vi "calibration.vi"(8 "error in (no error)":errorcluster, 10 "Pram_calib In":T1, 11 "Spectrum In":i64[](array[numeric])) -> (0 "Error Out":errorcluster, 1 "set max":cluster{"Channels":dbl[], "Intensity":dbl[]}, 2 "Param Calibrazione":T1, 3 "Spectrum Out":T3)   [LabVIEW 2023]
uses:
  control/calib.ctl
  control/param_calibrazione.ctl
  <vilib>/Analysis/1siggen.llb/Ramp Pattern by Samples.vi
  <vilib>/Utility/file.llb/Read Delimited Spreadsheet (string).vi
  control/global name path.vi
  <vilib>/Utility/file.llb/Write Delimited Spreadsheet (DBL).vi
  <vilib>/Utility/file.llb/Read Delimited Spreadsheet (DBL).vi
  queue/Front Panel Message Queue.lvlib
  <vilib>/Analysis/NI_AALBase.lvlib
panel:
  in  "load_spct":bool
  in  "save_spct":bool
  out "Load Param Calib":T1
  in  "load_param":bool
  in  "save_param":bool
  out "peaks found":i32
  out "Spectrum Init":T2(graph)
  in  "side points":i32=19
  in  "polynomial order":i32=9
  in  "Max Channel":i32=5800
  in  "Min Channel":i32=500
  in  "width":i32=60 min=3
  in  "threshold":dbl=50.0 format="%0.2f"
  out "Spectrum Calibrated":cluster{dbl[], dbl[]}(graph)
  in  "list_peak_energies":string[][](array[string])
  out "Calibration":cluster{dbl[], dbl[]}[](graph)
  in  "List Calibration":T4[](array[typedef]) {"Select Line" items=["Ka1", "Ka2", "Kb1", "La1", "La2", "Lb1", "Lb2", "Lg1"]; "Select Element" items=["Li", "Be", "B", "C", "N", "O", "F", "Ne", "Na", "Mg", "Al", "Si", "P", "S", "Cl", "Ar", "K", "Ca", "Sc", "Ti", "V", "Cr", "Mn", "Fe", "Co", "Ni", "Cu", "Zn", "Ga", "Ge", "As", "Se", "Br", "Kr", "Rb", "Sr", "Y", "Zr", "Nb", "Mo", "Tc", "Ru", "Rh", "Pd", "Ag", "Cd", "In", "Sn", "Sb", "Te", "I", "Xe", "Cs", "Ba", "La", "Ce", "Pr", "Nd", "Pm", "Sm", "Eu", "Gd", "Tb", "Dy", "Ho", "Er", "Tm", "Yb", "Lu", "Hf", "Ta", "W", "Re", "Os", "Ir", "Pt", "Au", "Hg", "Tl", "Pb", "Bi", "Po", "At", "Rn", "Fr", "Ra", "Ac", "Th", "Pa", "U", "Np", "Pu", "Am"]}
  in  "back":bool
  out "Spectrum Analyzed":cluster{"Channels":dbl[], "Intensity":dbl[]}[](graph)
  in  "smooth":bool
  in  "peak":bool
  in  "Stop Button":bool
  in  "Select Line":u16(ring) items=["Ka1", "Ka2", "Kb1", "La1", "La2", "Lb1", "Lb2", "Lg1"]
  in  "Select Element":u16(ring) items=["Li", "Be", "B", "C", "N", "O", "F", "Ne", "Na", "Mg", "Al", "Si", "P", "S", "Cl", "Ar", "K", "Ca", "Sc", "Ti", "V", "Cr", "Mn", "Fe", "Co", "Ni", "Cu", "Zn", "Ga", "Ge", "As", "Se", "Br", "Kr", "Rb", "Sr", "Y", "Zr", "Nb", "Mo", "Tc", "Ru", "Rh", "Pd", "Ag", "Cd", "In", "Sn", "Sb", "Te", "I", "Xe", "Cs", "Ba", "La", "Ce", "Pr", "Nd", "Pm", "Sm", "Eu", "Gd", "Tb", "Dy", "Ho", "Er", "Tm", "Yb", "Lu", "Hf", "Ta", "W", "Re", "Os", "Ir", "Pt", "Au", "Hg", "Tl", "Pb", "Bi", "Po", "At", "Rn", "Fr", "Ra", "Ac", "Th", "Pa", "U", "Np", "Pu", "Am"]
  # "Smooth Parameters"
  # "Search Peak Parameter"
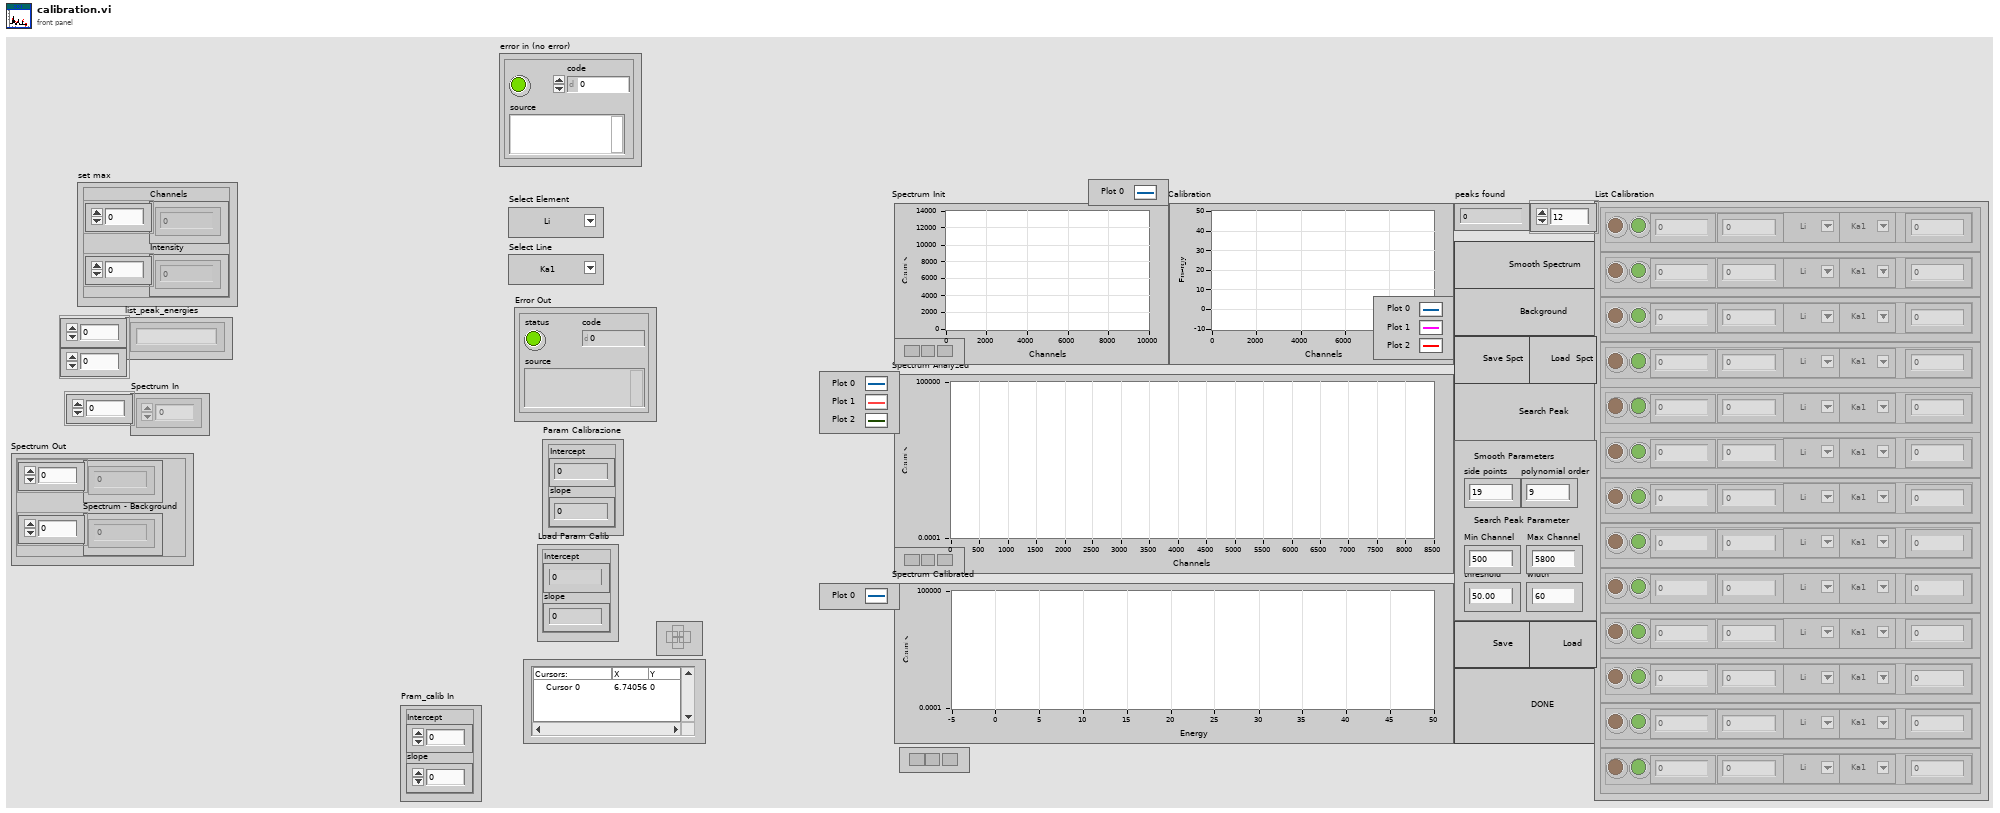
[diagram p1: front panel]
types:
  T1 = typedef "param_calibrazione.ctl" = cluster{"Intercept":dbl, "slope":dbl}
  T2 = cluster{"Ramp Pattern":dbl[], "Spectrum In":i64[]}
  T3 = cluster{"Array":dbl[], "Spectrum - Background":dbl[]}
  T4 = typedef "calib.ctl" = cluster{"select":bool, "Position":dbl, "Select Element":u16, "Select Line":u16, "Intensity":dbl, "Energy":dbl, "best":bool}
  T5 = typedef "Front Panel Message Queue.lvlib/Calibrazione Message Queues.ctl" = cluster{"Main":refnum<queue>, "Data":refnum<queue>}
  T6 = cluster{"Position":dbl[], "Intensity":dbl[], "Energy":dbl[]}
  T7 = cluster{"Ramp Pattern":dbl[], "Smoothed Spectrum":dbl[]}
  T8 = cluster{"Ramp Pattern":dbl[], "Spectrum - Background":dbl[]}
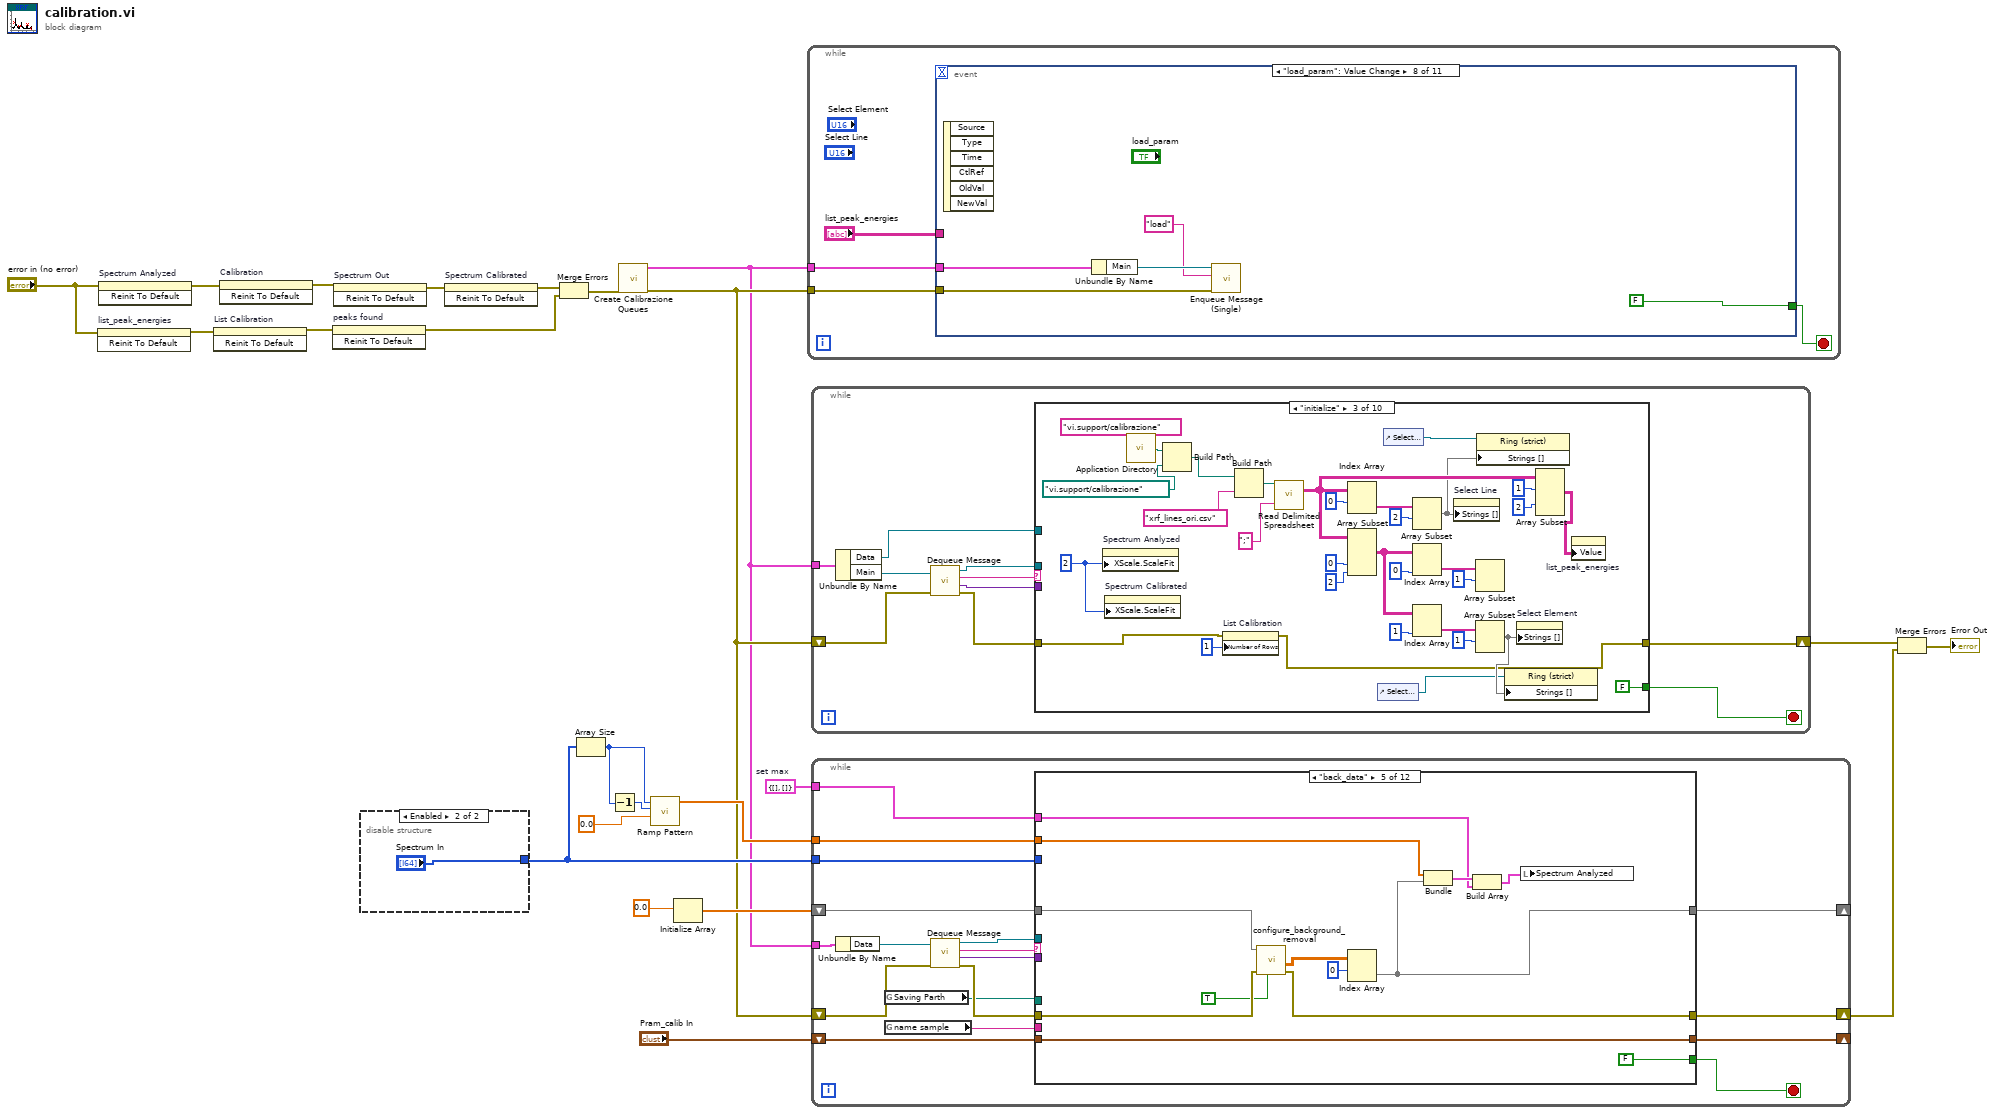
[diagram p0: block diagram]
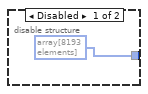
[diagram p2: hidden frame]
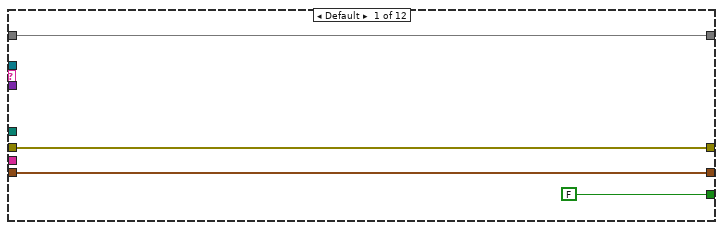
[diagram p3: hidden frame]
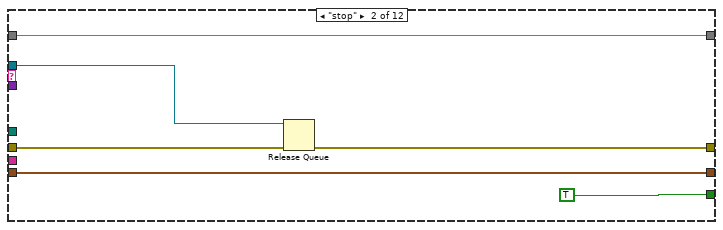
[diagram p4: hidden frame]
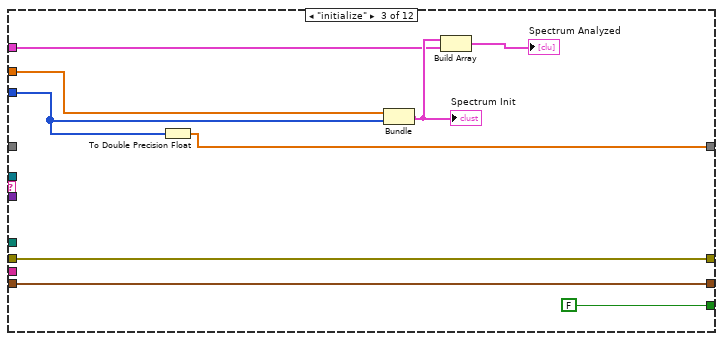
[diagram p5: hidden frame]
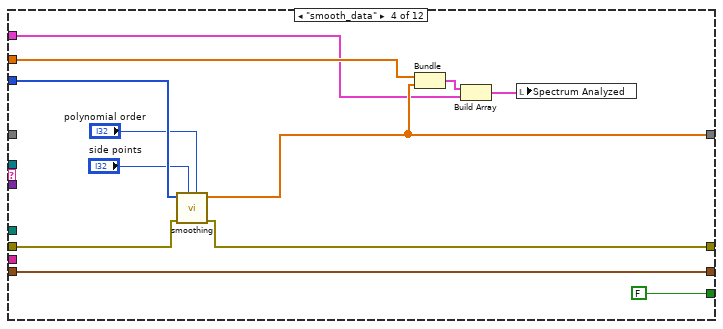
[diagram p6: hidden frame]
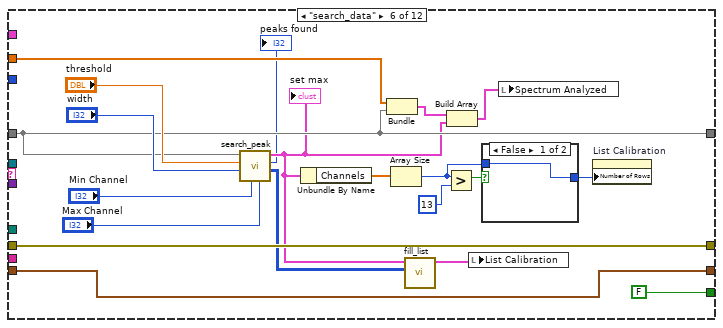
[diagram p7: hidden frame]
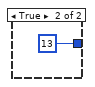
[diagram p8: hidden frame]
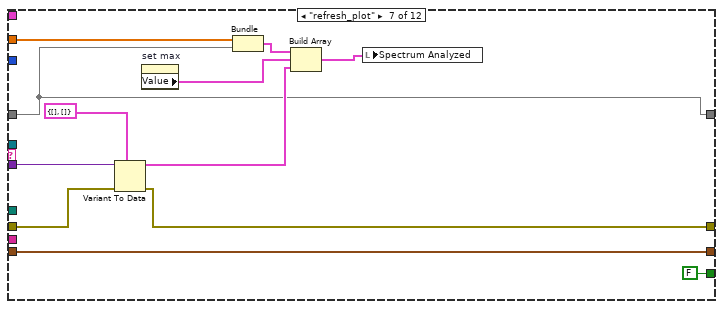
[diagram p9: hidden frame]
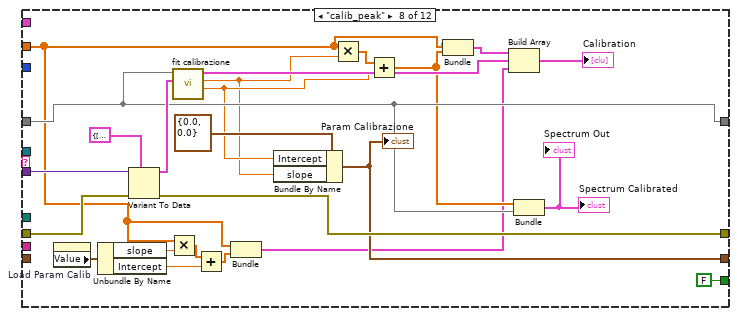
[diagram p10: hidden frame]
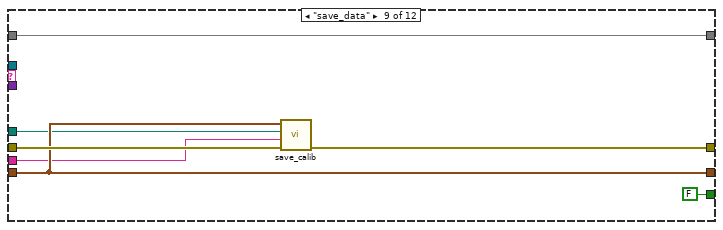
[diagram p11: hidden frame]
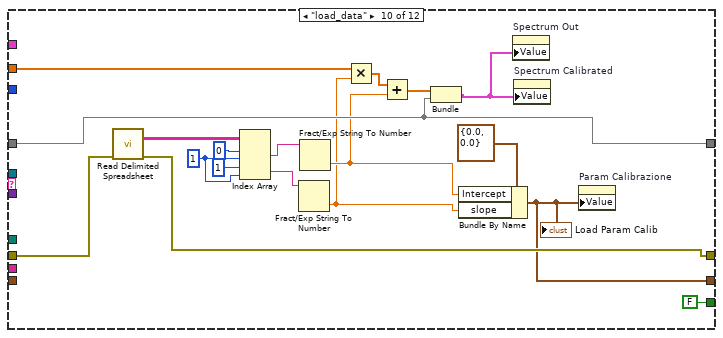
[diagram p12: hidden frame]
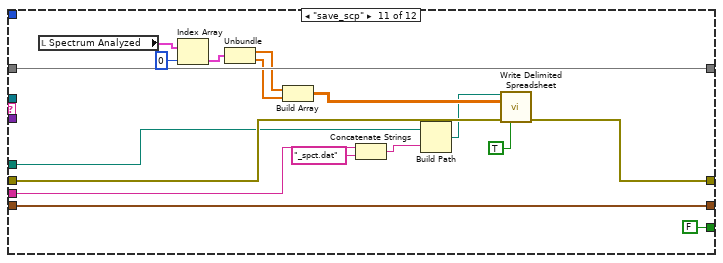
[diagram p13: hidden frame]
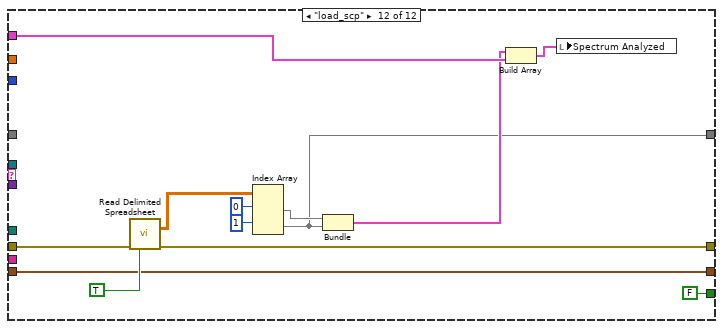
[diagram p14: hidden frame]
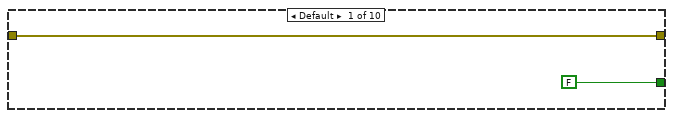
[diagram p15: hidden frame]
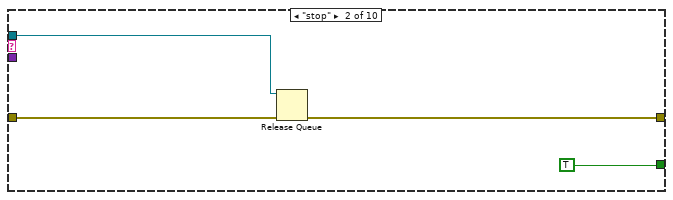
[diagram p16: hidden frame]
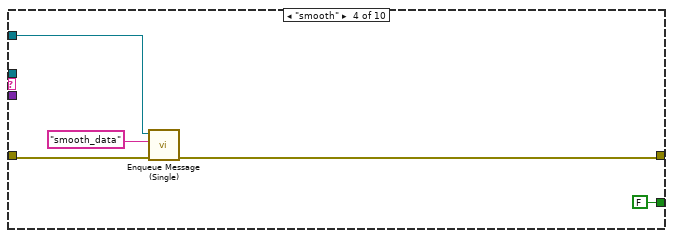
[diagram p17: hidden frame]
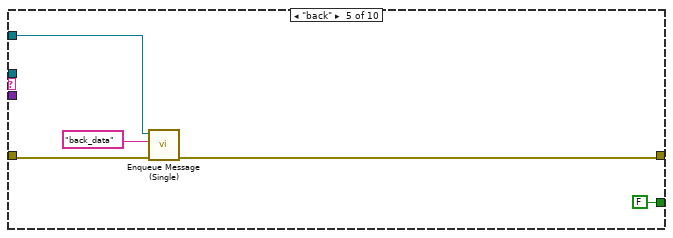
[diagram p18: hidden frame]
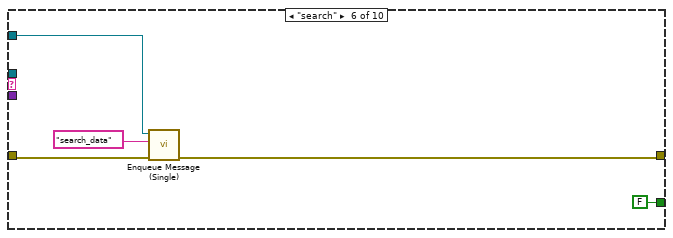
[diagram p19: hidden frame]
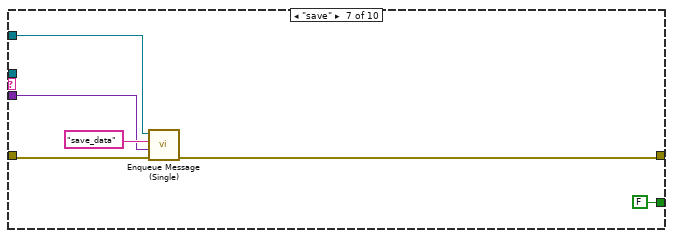
[diagram p20: hidden frame]
diagram:
  w16 = cluster{"Channels":dbl[], "Intensity":dbl[]} {"Channels"=[], "Intensity"=[]}  # set max
  n1 = invoke on="list_peak_energies" class="Arr (strict)" method="Reinit To Default"(error in="error in (no error)") -> (error out=w11:errorcluster)  [unwired: 2 in, 2 out]
  n2 = invoke on="Spectrum Analyzed" class="XYGraph (strict)" method="Reinit To Default"(error in="error in (no error)") -> (error out=w13:errorcluster)  [unwired: 2 in, 2 out]
  n3 = invoke on="List Calibration" class="Arr (strict)" method="Reinit To Default"(error in=w11) -> (error out=w9:errorcluster)  [unwired: 2 in, 2 out]
  n4 = invoke on="Calibration" class="XYGraph (strict)" method="Reinit To Default"(error in=w13) -> (error out=w14:errorcluster)  [unwired: 2 in, 2 out]
  n5 = invoke on="peaks found" class="DigNum (strict)" method="Reinit To Default"(error in=w9) -> (error out=w7:errorcluster)  [unwired: 2 in, 2 out]
  n6 = invoke on="Spectrum Out" class="Clust (strict)" method="Reinit To Default"(error in=w14) -> (error out=w12:errorcluster)  [unwired: 2 in, 2 out]
  n7 = disable-structure shown="Enabled" {
    disable-tunnel: [i64[] array[8193 elements] ("subarray") "Spectrum In"] -> w17
    frame Disabled {
    }
    frame Enabled {
    }
  }
  n8 = invoke on="Spectrum Calibrated" class="XYGraph (strict)" method="Reinit To Default"(error in=w12) -> (error out=w8:errorcluster)  [unwired: 2 in, 2 out]
  n9 = Merge Errors(w8, w7) -> (w6:errorcluster)
  n10 = Array Size(array=w17) -> (size(s)=w19:i32)
  n11 = Decrement(x=w19) -> (x-1=w20:i32)
  n12 = call "Create Calibrazione Queues.vi"("error in (no error)"=w6) -> ("error out"=w15:errorcluster, "Message Queues"=w1:T5)  [unwired: 9 in]
  n13 = call-poly <vilib>:"Ramp Pattern.vi"("start"=0.0, "end"=w20, "samples"=w19) -> ("Ramp Pattern"=w18:dbl[])  [unwired: 7 in, 1 out]
  n14 = Initialize Array(0.0) -> (w22:dbl[])  [unwired: 1 in]
  n15 = while {
    tunnel: w1 -> [w29]
    tunnel: w15 -> [w27]
    stop <- w28 stop-if-true
    n16 = event shown="[7] \"load_param\": Value Change" {
      selector: _ -> [_ _ _ _ _ _ _ _ _ _ _]
      dyn-events: _ -> [_ _ _ _ _ _ _ _ _ _ _]
      timeout: _ -> [_ _ _ _ _ _ _ _ _ _ _]
      tunnel: w29 -> [_ w37 w42 w48 w68 w87 w92 w97 w102 w107 _]
      tunnel: [FALSE TRUE FALSE FALSE FALSE FALSE FALSE FALSE FALSE FALSE FALSE] -> w28
      tunnel: w27 -> [_ w35 w43 w46 w69 w85 w90 w95 w100 w105 w109]
      tunnel: "list_peak_energies" -> [_ _ _ _ w52 _ _ _ _ _ _]
      event Timeout {
        n17 = event-data() -> ()  [unwired: 1 in, 3 out]
      }
      event "Stop Button": Value Change {
        w31 = "stop"
        w36 = TRUE
        n18 = event-data() -> ()  [unwired: 1 in, 6 out]
        n19 = Unbundle By Name(w37) -> ("Main"=w33:refnum<queue>, "Data"=w32:refnum<queue>)
        n20 = call "Enqueue Message (Single).vi"("Priority Message? (F)"=w36, "error in (no error)"=w35, "Message"=w31, "Message Queue"=w33) -> ("error out"=w34:errorcluster)  [unwired: 6 in, 1 out]
        n21 = call "Enqueue Message (Single).vi"("Priority Message? (F)"=w36, "error in (no error)"=w34, "Message"=w31, "Message Queue"=w32) -> ()  [unwired: 6 in, 2 out]
      }
      event "smooth": Value Change {
        n22 = event-data() -> ()  [unwired: 1 in, 6 out]
        n23 = Unbundle By Name(w42) -> ("Main"=w41:refnum<queue>)
        n24 = call "Enqueue Message (Single).vi"("error in (no error)"=w43, "Message"="smooth", "Message Queue"=w41) -> ()  [unwired: 7 in, 2 out]
      }
      event "peak": Value Change {
        n25 = event-data() -> ()  [unwired: 1 in, 6 out]
        n26 = Unbundle By Name(w48) -> ("Main"=w47:refnum<queue>)
        n27 = call "Enqueue Message (Single).vi"("error in (no error)"=w46, "Message"="search", "Message Queue"=w47) -> ()  [unwired: 7 in, 2 out]
      }
      event "List Calibration": Value Change {
        n28 = event-data() -> ("NewVal"=w51:T4[])  [unwired: 1 in, 5 out]
        n29 = Unbundle By Name(w68) -> ("Data"=w65:refnum<queue>)
        n30 = call "energy_list.vi"("list_peak_energies"=w52, "List Calibration"=w51) -> ("Check"=w49:bool[], "to calibrate"=w56:T6, "List Calibration Out"=w50:T4[])  [unwired: 7 in]
        n31 = property on="List Calibration" class="Arr (strict)"("Value"=w50) -> ()  [unwired: 2 in, 2 out]
        n32 = Unbundle By Name(w56) -> ("Position"=w53:dbl[], "Intensity"=w54:dbl[], "Energy"=w55:dbl[])
        n33 = Search 1D Array(1D array=w49, element=TRUE) -> (index of element=w58:i32)  [unwired: 1 in]
        n34 = Array Size(array=w55) -> (size(s)=w62:i32)
        n35 = Greater Or Equal To 0?(x=w58) -> (x >= 0?=w57:bool)
        n36 = Greater?(x=w62, y=1) -> (0:w60:bool)
        n37 = Bundle("Position"=w53, "Intensity"=w54) -> (w67:cluster{"Position":dbl[], "Intensity":dbl[]})  [unwired: 1 in]
        n38 = To Variant(anything=w67) -> (Variant=w66:variant)
        n39 = Bundle("Position"=w53, "Intensity"=w54, "Energy"=w55) -> (w64:T6)  [unwired: 1 in]
        n40 = To Variant(anything=w64) -> (Variant=w63:variant)
        n41 = case shown="True" w57 {
          tunnel: w69 -> [_ w78]
          tunnel: w66 -> [_ w75]
          tunnel: w65 -> [_ w74]
          tunnel: w63 -> [_ w72]
          tunnel: w60 -> [_ w71]
          frame False {
          }
          frame True {
            n42 = call "Enqueue Message (Single).vi"("error in (no error)"=w78, "Message Data"=w75, "Message"="refresh_plot", "Message Queue"=w74) -> ("error out"=w76:errorcluster, "dup Message Queue"=w73:refnum<queue>)  [unwired: 6 in]
            n43 = case shown="True" w71 {
              tunnel: w76 -> [_ w82]
              tunnel: w73 -> [_ w80]
              tunnel: w72 -> [_ w79]
              frame False {
              }
              frame True {
                n44 = call "Enqueue Message (Single).vi"("error in (no error)"=w82, "Message Data"=w79, "Message"="calib_peak", "Message Queue"=w80) -> ()  [unwired: 6 in, 2 out]
              }
            }
          }
        }
      }
      event "back": Value Change {
        n45 = event-data() -> ()  [unwired: 1 in, 6 out]
        n46 = Unbundle By Name(w87) -> ("Main"=w86:refnum<queue>)
        n47 = call "Enqueue Message (Single).vi"("error in (no error)"=w85, "Message"="back", "Message Queue"=w86) -> ()  [unwired: 7 in, 2 out]
      }
      event "save_param": Value Change {
        n48 = event-data() -> ()  [unwired: 1 in, 6 out]
        n49 = Unbundle By Name(w92) -> ("Main"=w91:refnum<queue>)
        n50 = call "Enqueue Message (Single).vi"("error in (no error)"=w90, "Message"="save", "Message Queue"=w91) -> ()  [unwired: 7 in, 2 out]
      }
      event "load_param": Value Change {
        n51 = event-data() -> ()  [unwired: 1 in, 6 out]
        n52 = Unbundle By Name(w97) -> ("Main"=w96:refnum<queue>)
        n53 = call "Enqueue Message (Single).vi"("error in (no error)"=w95, "Message"="load", "Message Queue"=w96) -> ()  [unwired: 7 in, 2 out]
      }
      event "save_spct": Value Change {
        n54 = event-data() -> ()  [unwired: 1 in, 6 out]
        n55 = Unbundle By Name(w102) -> ("Main"=w101:refnum<queue>)
        n56 = call "Enqueue Message (Single).vi"("error in (no error)"=w100, "Message"="save_scp", "Message Queue"=w101) -> ()  [unwired: 7 in, 2 out]
      }
      event "load_spct": Value Change {
        n57 = event-data() -> ()  [unwired: 1 in, 6 out]
        n58 = Unbundle By Name(w107) -> ("Main"=w106:refnum<queue>)
        n59 = call "Enqueue Message (Single).vi"("error in (no error)"=w105, "Message"="load_scp", "Message Queue"=w106) -> ()  [unwired: 7 in, 2 out]
      }
      event "Spectrum Calibrated": Mouse Up {
        w110 = u32 0 ("Active Plot")
        n60 = event-data() -> ()  [unwired: 1 in, 8 out]
        n61 = property on="Spectrum Calibrated" class="XYGraph (strict)"(error in=w109, "Active Plot"=w110, "Active Cursor"=w110) -> ("Cursor.Cursor X"=w108:dbl)  [unwired: 1 in, 2 out]
        n62 = call "list_peak.vi"("Position Energy"=w108) -> ()  [unwired: 11 in]
      }
    }
  }
  n63 = while {
    shift-right: [w117] -> w5
    shift-left: w15 -> [w120]
    tunnel: w1 -> [w112]
    stop <- w116 stop-if-true
    n64 = Unbundle By Name(w112) -> ("Data"=w114:refnum<queue>, "Main"=w121:refnum<queue>)
    n65 = call "Dequeue Message.vi"("error in (no error)"=w120, "Message Queue"=w121) -> ("error out"=w119:errorcluster, "Message Data"=w113:variant, "Message"=w118:string, "dup Message Queue"=w115:refnum<queue>)  [unwired: 5 in, 1 out]
    n66 = case shown="\"initialize\"" w118 {
      tunnel: w119 -> [w123 w126 w129 w162 w167 w172 w178 w183 w188 w193]
      tunnel: [w123 w125 w131 w161 w166 w171 w177 w182 w187 w192] -> w117
      tunnel: [FALSE TRUE FALSE FALSE FALSE FALSE FALSE FALSE FALSE FALSE] -> w116
      tunnel: w115 -> [_ w124 _ _ _ _ _ _ _ _]
      tunnel: w114 -> [_ _ _ w160 w165 w170 w176 w181 w186 w191]
      tunnel: w113 -> [_ _ _ _ _ _ w174 _ _ _]
      frame Default {
      }
      frame "stop" {
        n67 = Release Queue(queue=w124, error in (no error)=w126) -> (error out=w125:errorcluster)  [unwired: 1 in, 2 out]
      }
      frame "initialize" {
        w128 = 2 ("Active X Scale")
        (unwired) "vi.support/calibrazione"
        n68 = property on="Spectrum Analyzed" class="XYGraph (strict)"("XScale.ScaleFit"=w128) -> ()  [unwired: 2 in, 2 out]
        n69 = property on="Spectrum Calibrated" class="XYGraph (strict)"("XScale.ScaleFit"=w128) -> ()  [unwired: 2 in, 2 out]
        n70 = call <vilib>:"Application Directory.vi"() -> ("Application Directory"=w140:path)
        n71 = Build Path(base path=w140, name or relative path=path "vi.support/calibrazione") -> (appended path=w139:path)
        n72 = property on="List Calibration" class="Arr (strict)"(error in=w129, "Number of Rows"=u32 1) -> (error out=w131:errorcluster)  [unwired: 1 in, 1 out]
        n73 = Build Path(base path=w139, name or relative path="xrf_lines_ori.csv") -> (appended path=w156:path)
        n74 = call-poly <vilib>:"Read Delimited Spreadsheet.vi"("file path (dialog if empty)"=w156, "delimiter (\\t)"=";" ("delimiter (\\t)")) -> ("all rows"=w143:string[][])  [unwired: 8 in, 5 out]
        n75 = Index Array(array=w143, index (row)=0) -> (element=w144:string[])  [unwired: 1 in]
        n76 = Array Subset(array=w143, index (col)=0 ("index"), length (col)=2 ("length")) -> (w149:string[][])  [unwired: 2 in]
        n77 = control-ref of="Select Element"() -> (w134:refnum<vi>)
        n78 = control-ref of="Select Line"() -> (w135:refnum<vi>)
        n79 = Array Subset(array=w144, index=2) -> (w136:string[])  [unwired: 1 in]
        n80 = Index Array(array=w149, index (col)=0 ("index (row)")) -> (element=w148:string[])  [unwired: 1 in]
        n81 = Index Array(array=w149, index (col)=1 ("index (row)")) -> (element=w146:string[])  [unwired: 1 in]
        n82 = property on="Select Line" class="Ring (strict)"("Strings []"=w136) -> ()  [unwired: 2 in, 2 out]
        n83 = Array Subset(array=w148, index=1) -> ()  [unwired: 1 in, 1 out]
        n84 = Array Subset(array=w146, index=1) -> (w137:string[])  [unwired: 1 in]
        n85 = property class="Ring (strict)"(reference=w135, "Strings []"=w136) -> ()  [unwired: 1 in, 2 out]
        n86 = property class="Ring (strict)"(reference=w134, "Strings []"=w137) -> ()  [unwired: 1 in, 2 out]
        n87 = property on="Select Element" class="Ring (strict)"("Strings []"=w137) -> ()  [unwired: 2 in, 2 out]
        n88 = Array Subset(array=w143, index (row)=1 ("index"), index (col)=2 ("index")) -> (w132:string[][])  [unwired: 2 in]
        n89 = property on="list_peak_energies" class="Arr (strict)"("Value"=w132) -> ()  [unwired: 2 in, 2 out]
      }
      frame "smooth" {
        n90 = call "Enqueue Message (Single).vi"("error in (no error)"=w162, "Message"="smooth_data", "Message Queue"=w160) -> ("error out"=w161:errorcluster)  [unwired: 7 in, 1 out]
      }
      frame "back" {
        n91 = call "Enqueue Message (Single).vi"("error in (no error)"=w167, "Message"="back_data", "Message Queue"=w165) -> ("error out"=w166:errorcluster)  [unwired: 7 in, 1 out]
      }
      frame "search" {
        n92 = call "Enqueue Message (Single).vi"("error in (no error)"=w172, "Message"="search_data", "Message Queue"=w170) -> ("error out"=w171:errorcluster)  [unwired: 7 in, 1 out]
      }
      frame "save" {
        n93 = call "Enqueue Message (Single).vi"("error in (no error)"=w178, "Message Data"=w174, "Message"="save_data", "Message Queue"=w176) -> ("error out"=w177:errorcluster)  [unwired: 6 in, 1 out]
      }
      frame "load" {
        n94 = call "Enqueue Message (Single).vi"("error in (no error)"=w183, "Message"="load_data", "Message Queue"=w181) -> ("error out"=w182:errorcluster)  [unwired: 7 in, 1 out]
      }
      frame "save_scp" {
        n95 = call "Enqueue Message (Single).vi"("error in (no error)"=w188, "Message"="save_scp", "Message Queue"=w186) -> ("error out"=w187:errorcluster)  [unwired: 7 in, 1 out]
      }
      frame "load_scp" {
        n96 = call "Enqueue Message (Single).vi"("error in (no error)"=w193, "Message"="load_scp", "Message Queue"=w191) -> ("error out"=w192:errorcluster)  [unwired: 7 in, 1 out]
      }
    }
  }
  n97 = while {
    shift-right: [w208] -> w4
    shift-left: w15 -> [w211]
    tunnel: w17 -> [w205]
    shift-right: [w202] -> _
    shift-left: w22 -> [w204]
    tunnel: w18 -> [w203]
    tunnel: w16 -> [w201]
    shift-right: [w199] -> _
    shift-left: "Pram_calib In" -> [w198]
    tunnel: w1 -> [w197]
    stop <- w207 stop-if-true
    n98 = Unbundle By Name(w197) -> ("Data"=w212:refnum<queue>)
    n99 = global read "global name path.vi" "Saving Parth"() -> (w196:path)
    n100 = global read "global name path.vi" "name sample"() -> (w195:string)
    n101 = call "Dequeue Message.vi"("error in (no error)"=w211, "Message Queue"=w212) -> ("error out"=w210:errorcluster, "Message Data"=w200:variant, "Message"=w209:string, "dup Message Queue"=w206:refnum<queue>)  [unwired: 5 in, 1 out]
    n102 = case shown="\"back_data\"" w209 {
      tunnel: w210 -> [w216 w221 w225 w242 w256 w271 w289 w313 w318 w338 w353 w366]
      tunnel: [w216 w220 w225 w241 w255 w271 w283 w312 w319 w323 w352 w363] -> w208
      tunnel: [FALSE TRUE FALSE FALSE FALSE FALSE FALSE FALSE FALSE FALSE FALSE FALSE] -> w207
      tunnel: w206 -> [_ w219 _ _ _ _ _ _ _ _ _ _]
      tunnel: w205 -> [_ _ w224 w243 _ _ _ _ _ _ _ _]
      tunnel: [w214 w218 w223 w237 w249 w269 w281 w304 w321 w328 w356 w357] -> w202
      tunnel: w204 -> [w214 w218 _ _ w251 w269 w281 w304 w321 w328 w356 _]
      tunnel: w203 -> [_ _ w230 w236 w248 w274 w288 w293 _ w332 _ _]
      tunnel: w201 -> [_ _ w227 w233 w245 _ _ _ _ _ _ w367]
      tunnel: w200 -> [_ _ _ _ _ _ w290 w314 _ _ _ _]
      tunnel: [w213 w217 w226 w232 w244 w257 w279 w298 w317 w322 w354 w364] -> w199
      tunnel: w198 -> [w213 w217 w226 w232 w244 w257 w279 _ w317 _ w354 w364]
      tunnel: w195 -> [_ _ _ _ _ _ _ _ w316 _ w342 _]
      tunnel: w196 -> [_ _ _ _ _ _ _ _ w315 _ w345 _]
      frame Default {
      }
      frame "stop" {
        n103 = Release Queue(queue=w219, error in (no error)=w221) -> (error out=w220:errorcluster)  [unwired: 1 in, 2 out]
      }
      frame "initialize" {
        n104 = To Double Precision Float(number=w224) -> (double precision float=w223:dbl[])
        n105 = Bundle("Ramp Pattern"=w230, "Spectrum In"=w224) -> (w229:T2)  [unwired: 1 in]
        "Spectrum Init" <- w229
        n106 = Build Array(w229, w227) -> (→"Spectrum Analyzed":cluster{"Channels":dbl[], "Intensity":dbl[]}[])
      }
      frame "smooth_data" {
        n107 = call "smoothing.vi"("polynomial order"="polynomial order", "side points"="side points", "Error In"=w242, "Spectrum"=w243) -> ("Error Out"=w241:errorcluster, "Smoothed Spectrum"=w237:dbl[])  [unwired: 6 in]
        n108 = Bundle("Ramp Pattern"=w236, "Smoothed Spectrum"=w237) -> (w234:T7)  [unwired: 1 in]
        n109 = Build Array(w234, w233) -> (w235:cluster{"Channels":dbl[], "Intensity":dbl[]}[])
        n110 = local write "Spectrum Analyzed"(w235) -> ()
      }
      frame "back_data" {
        n111 = call "configure_background_removal.vi"("Is ASCII File?"=TRUE, "error in (no error)"=w256, "Spectrum In"=w251) -> ("error out"=w255:errorcluster, "Spectrum - Background"=w253:dbl[][])  [unwired: 5 in, 2 out]
        n112 = Index Array(array=w253, index (row)=0) -> (element=w249:dbl[])  [unwired: 1 in]
        n113 = Bundle("Ramp Pattern"=w248, "Spectrum - Background"=w249) -> (w247:T8)  [unwired: 1 in]
        n114 = Build Array(w247, w245) -> (w246:cluster{"Channels":dbl[], "Intensity":dbl[]}[])
        n115 = local write "Spectrum Analyzed"(w246) -> ()
      }
      frame "search_data" {
        n116 = call "search_peak.vi"("Max Channel"="Max Channel", "Min Channel"="Min Channel", "width"="width", "threshold"="threshold", "Spectrum"=w269) -> ("Best 8"=w258:i32[][], "peaks found"=→"peaks found":i32, "set max"=w265:cluster{"Channels":dbl[], "Intensity":dbl[]})  [unwired: 4 in]
        "set max" <- w265
        n117 = Unbundle By Name(w265) -> ("Channels"=w266:dbl[])
        n118 = Bundle("Ramp Pattern"=w274, "all rows"=w269) -> (w275:cluster{"Ramp Pattern":dbl[], "all rows":dbl[]})  [unwired: 1 in]
        n119 = Array Size(array=w266) -> (size(s)=w260:i32)
        n120 = call "fill_list.vi"("Best 8"=w258, "set max"=w265) -> ("List Calibration"=w264:T4[])  [unwired: 9 in]
        n121 = Greater?(x=w260, y=13) -> (0:w261:bool)
        n122 = Build Array(w275, w265) -> (w270:cluster{"Channels":dbl[], "Intensity":dbl[]}[])
        n123 = local write "List Calibration"(w264) -> ()
        n124 = case shown="False" w261 {
          tunnel: w260 -> [w277 _]
          tunnel: [w277 13 ("y")] -> w259
          frame False {
          }
          frame True {
          }
        }
        n125 = local write "Spectrum Analyzed"(w270) -> ()
        n126 = property on="List Calibration" class="Arr (strict)"("Number of Rows"=w259) -> ()  [unwired: 2 in, 2 out]
      }
      frame "refresh_plot" {
        n127 = Variant To Data(error in=w289, type=cluster{dbl[], dbl[]} {[], []} ("output cluster"), Variant=w290) -> (data=w284:cluster{dbl[], dbl[]}, error out=w283:errorcluster)
        n128 = property on="set max" class="Clust (strict)"() -> ("Value"=w285:cluster{"Channels":dbl[], "Intensity":dbl[]})  [unwired: 2 in, 2 out]
        n129 = Bundle("Ramp Pattern"=w288, "all rows"=w281) -> (w286:cluster{"Ramp Pattern":dbl[], "all rows":dbl[]})  [unwired: 1 in]
        n130 = Build Array(w286, w285, w284) -> (w280:cluster{"Channels":dbl[], "Intensity":dbl[]}[])
        n131 = local write "Spectrum Analyzed"(w280) -> ()
      }
      frame "calib_peak" {
        n132 = property on="Load Param Calib" class="Clust (strict)"() -> ("Value"=w291:T1)  [unwired: 2 in, 2 out]
        n133 = Unbundle By Name(w291) -> ("slope"=w296:dbl, "Intercept"=w295:dbl)
        n134 = Variant To Data(error in=w313, type=cluster{dbl[], dbl[], dbl[]} {[], [], []} ("output cluster"), Variant=w314) -> (data=w306:cluster{dbl[], dbl[], dbl[]}, error out=w312:errorcluster)
        n135 = Multiply(x=w293, y=w296) -> (x*y=w297:dbl[])
        n136 = call "fit calibrazione.vi"("data"=w306, "Spectrum - Background"=w304) -> ("intercept"=w300:dbl, "slope"=w299:dbl, "Ch_Ene"=w305:cluster{"Array":dbl[], "Array":dbl[]})  [unwired: 7 in]
        n137 = Add(x=w297, y=w295) -> (x+y=w294:dbl[])
        n138 = Bundle("Ramp Pattern"=w293, w294) -> (w292:cluster{"Ramp Pattern":dbl[], dbl[]})  [unwired: 1 in]
        n139 = Bundle By Name(cluster=T1 {"Intercept"=0.0, "slope"=0.0} ("param_calib"), "Intercept"=w300, "slope"=w299) -> (w298:T1)
        "Param Calibrazione" <- w298
        n140 = Multiply(x=w293, y=w299) -> (x*y=w308:dbl[])
        n141 = Add(x=w308, y=w300) -> (x+y=w303:dbl[])
        n142 = Bundle("Ramp Pattern"=w293, w303) -> (w307:cluster{"Ramp Pattern":dbl[], dbl[]})  [unwired: 1 in]
        n143 = Build Array(w307, w305, w292) -> (→"Calibration":cluster{"Ramp Pattern":dbl[], "Array":dbl[]}[])
        n144 = Bundle(w303, "all rows"=w304) -> (→"Spectrum Calibrated" →"Spectrum Out":cluster{dbl[], "all rows":dbl[]})  [unwired: 1 in]
      }
      frame "save_data" {
        n145 = call "save_calib.vi"("error in (no error)"=w318, "name sample"=w316, "Save Path"=w315, "Param. Calib"=w317) -> ("error out"=w319:errorcluster)  [unwired: 7 in]
      }
      frame "load_data" {
        w334 = 1 ("disabled index (col)")
        n146 = call-poly <vilib>:"Read Delimited Spreadsheet.vi"("error in (no error)"=w338) -> ("all rows"=w337:string[][], "error out"=w323:errorcluster)  [unwired: 9 in, 4 out]
        n147 = Index Array(array=w337, index (row) #1=0 ("index (row)"), index (col) #1=w334, index (row) #2=1 ("index (row)"), index (col) #2=w334) -> (element #1=w331:string, element #2=w330:string)
        n148 = Fract/Exp String To Number(string=w330) -> (number=w324:dbl)  [unwired: 3 in, 1 out]
        n149 = Fract/Exp String To Number(string=w331) -> (number=w325:dbl)  [unwired: 3 in, 1 out]
        n150 = Multiply(x=w332, y=w324) -> (x*y=w333:dbl[])
        n151 = Add(x=w333, y=w325) -> (x+y=w329:dbl[])
        n152 = Bundle(w329, "all rows"=w328) -> (w327:cluster{dbl[], "all rows":dbl[]})  [unwired: 1 in]
        n153 = Bundle By Name(cluster=T1 {"Intercept"=0.0, "slope"=0.0} ("param_calib"), "Intercept"=w325, "slope"=w324) -> (w322:T1)
        "Load Param Calib" <- w322
        n154 = property on="Spectrum Out" class="Clust (strict)"("Value"=w327) -> ()  [unwired: 2 in, 2 out]
        n155 = property on="Spectrum Calibrated" class="XYGraph (strict)"("Value"=w327) -> ()  [unwired: 2 in, 2 out]
        n156 = property on="Param Calibrazione" class="Clust (strict)"("Value"=w322) -> ()  [unwired: 2 in, 2 out]
      }
      frame "save_scp" {
        n157 = local read "Spectrum Analyzed"() -> (w351:cluster{"Channels":dbl[], "Intensity":dbl[]}[])
        n158 = Index Array(array=w351, index=0) -> (element=w349:cluster{"Channels":dbl[], "Intensity":dbl[]})
        n159 = Unbundle(w349) -> ("Channels"=w348:dbl[], "Intensity"=w347:dbl[])
        n160 = Build Array(w348, w347) -> (w346:dbl[][])
        n161 = Concatenate Strings(w342, "_spct.dat" ("string")) -> (w340:string)
        n162 = Build Path(base path=w345, name or relative path=w340) -> (appended path=w343:path)
        n163 = call-poly <vilib>:"Write Delimited Spreadsheet.vi"("file path (dialog if empty)"=w343, "2D data"=w346, "error in (no error)"=w353, "transpose? (no:F)"=TRUE) -> ("error out"=w352:errorcluster)  [unwired: 10 in, 1 out]
      }
      frame "load_scp" {
        n164 = call-poly <vilib>:"Read Delimited Spreadsheet.vi"("error in (no error)"=w366, "transpose? (F)"=TRUE) -> ("all rows"=w362:dbl[][], "error out"=w363:errorcluster)  [unwired: 8 in, 4 out]
        n165 = Index Array(array=w362, index (row) #1=0 ("index (row)"), index (row) #2=1 ("index (row)")) -> (element #1=w359:dbl[], element #2=w357:dbl[])  [unwired: 2 in]
        n166 = Bundle("all rows"=w359, "all rows"=w357) -> (w358:cluster{"all rows":dbl[], "all rows":dbl[]})  [unwired: 1 in]
        n167 = Build Array(w358, w367) -> (w368:cluster{"Channels":dbl[], "Intensity":dbl[]}[])
        n168 = local write "Spectrum Analyzed"(w368) -> ()
      }
    }
  }
  n169 = Merge Errors(w5, w4) -> (→"Error Out":errorcluster)
